vi "Search for Waveform.vi"(9 "NI_ChannelName":string, 10 "Waveforms":waveform(dbl)[](array[waveform])) -> (1 "Waveform Found?":bool, 2 "Waveform":waveform(dbl))   [LabVIEW 2021]
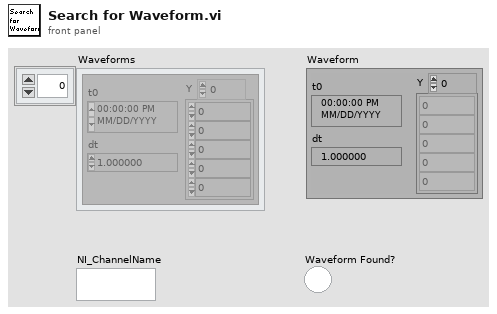
[diagram p1: front panel]
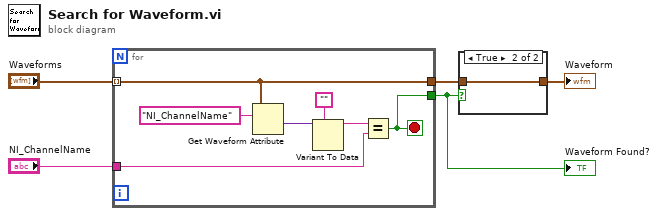
[diagram p0: block diagram]
diagram:
  n1 = for {
    tunnel: "Waveforms" -> [w10] mode=indexing
    tunnel: [w10] -> w4
    tunnel: [w8] -> w5
    tunnel: "NI_ChannelName" -> [w7]
    stop <- w8 stop-if-true
    n2 = Get Waveform Attribute(6:"NI_ChannelName" ("name"), 7:w10) -> (1:w11:variant)  [unwired: 2 in, 3 out]
    n3 = Variant To Data(type="", Variant=w11) -> (data=w9:string)  [unwired: 1 in, 1 out]
    n4 = Equal?(x=w9, y=w7) -> (x = y?=w8:bool)
  }
  "Waveform Found?" <- w5
  n5 = case shown="True" w5 {
    tunnel: [_ w13] -> w1
    tunnel: w4 -> [_ w13]
    frame False {
    }
    frame True {
    }
  }
  "Waveform" <- w1
